vi "Add User.vi"(8 "error in (no error)":errorcluster, 11 "TestCase in":refnum<class "Add User.lvclass">=refnum) -> (0 "error out":errorcluster, 3 "TestCase out":refnum<class "Add User.lvclass">)   [LabVIEW 2017, in "Add User.lvclass"]
uses:
  Add User.lvclass
  Source/User Configuration Manager Ref/By Ref.lvlib
  Source/iUser Configuration Manager/iUser Configuration Manager.lvclass
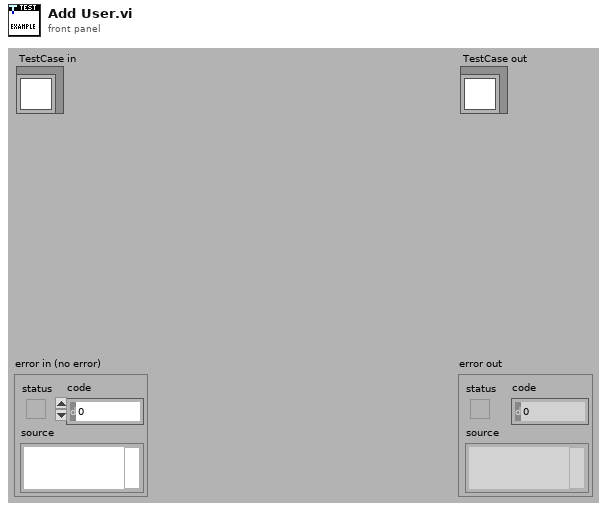
[diagram p1: front panel]
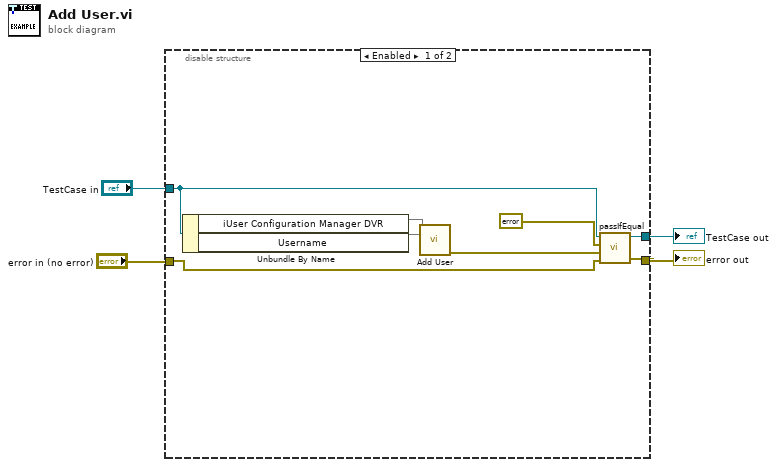
[diagram p0: block diagram]
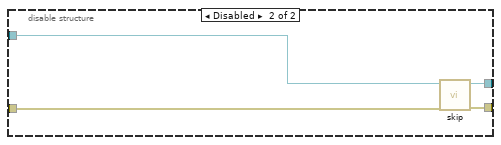
[diagram p2: hidden frame]
diagram:
  n1 = disable-structure "This diagram is for convenience to enable skipping a test easily (enable 'Skip' case)" shown="Enabled" {
    disable-tunnel: "TestCase in" -> [w10 w16]
    disable-tunnel: [w12 w14] -> w1
    disable-tunnel: [w11 w15] -> w3
    disable-tunnel: "error in (no error)" -> [w5 w13]
    frame Enabled {
      n2 = Unbundle By Name(w10) -> ("iUser Configuration Manager DVR"=w9, "Username"=w8)
      n3 = call "Add User.vi"("iUser Configuration Manager DVR"=w9, "Username"=w8) -> ("error out"=w7:errorcluster)  [unwired: 11 in, 2 out]
      n4 = call-dynamic "passIfEqual.vi"("error in (no error)"=w5, "y"=w7, "x"=errorcluster {"status"=FALSE, "code"=0, "source"=""} ("error out"), "TestCase in"=w10) -> ("error out"=w11:errorcluster, "TestCase out"=w12:refnum<class "Add User.lvclass">)  [unwired: 6 in]
    }
    frame Disabled {
      n5 = call <vilib>:"skip.vi"("error in (no error)"=w13, "TestCase in"=w16) -> ("error out"=w15:errorcluster, "TestCase out"=w14:refnum<class "Add User.lvclass">)  [unwired: 8 in]
    }
  }
  "error out" <- w3
  "TestCase out" <- w1
